vi "Get Tag.vi"(8 "Error In":errorcluster, 11 "Display Element In":refnum<class "Display Element.lvclass">) -> (0 "Error Out":errorcluster, 2 "Tag":string, 3 "Display Element Out":refnum<class "Display Element.lvclass">)   [LabVIEW 2019, in "Display Element.lvclass"]
uses:
  Display Element.lvclass
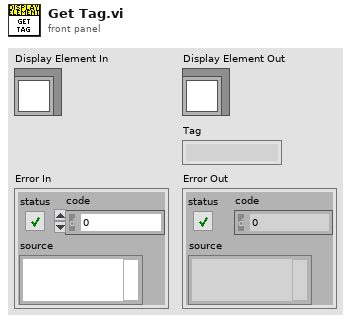
[diagram p1: front panel]
types:
  T1 = typedef "Display Element.lvclass/Data.ctl" = cluster{"Color":u32, "Layer":u32, "Tag":string, "Position":T2, "Force":T2, "Delete If Outside Bounds":bool}
  T2 = typedef "Display Element.lvclass/Vector.ctl" = cluster{"X":i32, "Y":i32}
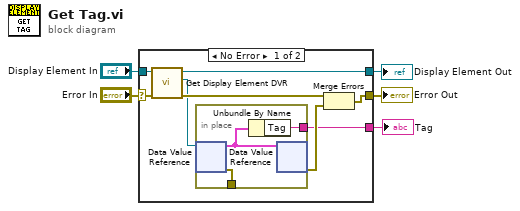
[diagram p0: block diagram]
diagram:
  n1 = case shown="No Error" "Error In" {
    selector: "Error In" -> [w9 w17]
    tunnel: [w11 w17] -> w4
    tunnel: [w8 w18] -> w2
    tunnel: "Display Element In" -> [w10 w18]
    tunnel: [w12 _] -> w1
    frame No Error {
      n2 = call "Get Display Element DVR.vi"("Error In"=w9, "Display Element In"=w10) -> ("Error Out"=w7:errorcluster, "DVR"=w6:refnum<data-value>, "Display Element Out"=w8:refnum<class "Display Element.lvclass">)  [unwired: 7 in]
      n3 = in-place {
        in-place-border: [w14] -> w12
        in-place-border: [w16] -> _
        n4 = in-place-dvr #1(w6) -> (w15:T1, w16:errorcluster)
        n5 = Unbundle By Name(w15) -> ("Tag"=w14:string)
        n6 = in-place-dvr #1(w15) -> (w13:errorcluster)  [unwired: 1 out]
      }
      n7 = Merge Errors(w7, w13) -> (w11:errorcluster)
    }
    frame Error {
    }
  }
  "Display Element Out" <- w2
  "Error Out" <- w4
  "Tag" <- w1
